vi "postCommandUserEvent.vi"(8 "error in (no error)":errorcluster, 10 "unsigned byte array":u8[](array[numeric]), 11 "DataListenerThisComponent in":refnum<class "DataListenerThisComponent.lvclass">) -> (0 "error out":errorcluster, 3 "DataListenerThisComponent out":refnum<class "DataListenerThisComponent.lvclass">)   [LabVIEW 2015, in "DataListenerThisComponent.lvclass"]
uses:
  DataListenerThisComponent.lvclass
  ComponentTemplateCore/ComponentModel/ComponentModel/DataListener/DataListener.lvclass/DataListener.ctl
  ComponentTemplateCore/ComponentModel/ComponentModel/CommandEvent/CommandEvent.lvclass/CommandEvent.ctl
  ComponentTemplateCore/ComponentModel/ComponentModel/CommandEvent/CommandEvent.lvclass
  ComponentTemplateCore/ComponentModel/ComponentModel/DataListener/DataListener.lvclass
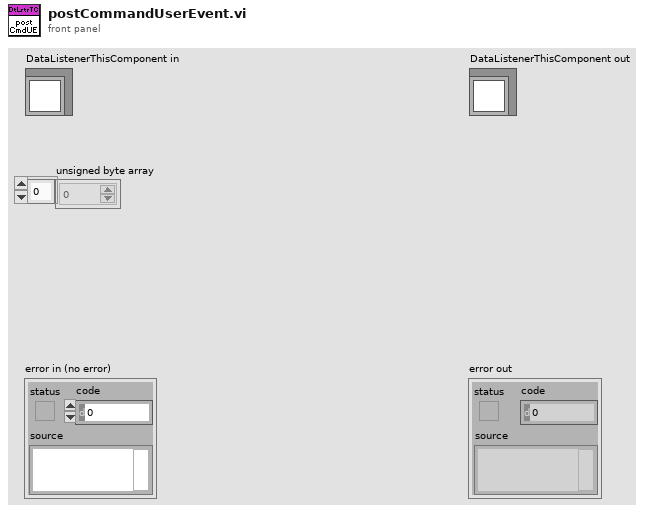
[diagram p1: front panel]
types:
  T1 = typedef "EXATypedefs.lvlib/CommandEvents.ctl" = cluster{"command":refnum<user-event>}
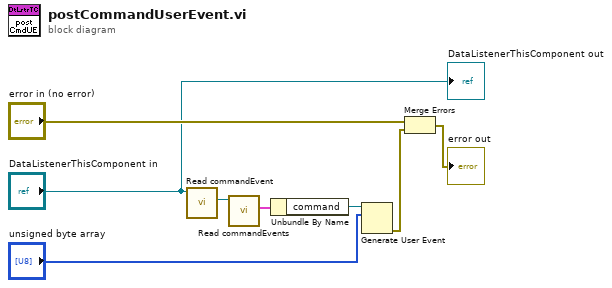
[diagram p0: block diagram]
diagram:
  n1 = call "Read commandEvent.vi"("DataListener in"="DataListenerThisComponent in") -> ("commandEvent"=w2:refnum<class "CommandEvent.lvclass">)  [unwired: 9 in, 1 out]
  n2 = call "Read commandEvents.vi"("CommandEvent in"=w2) -> ("CommandEvents"=w1:T1)  [unwired: 9 in, 1 out]
  n3 = Unbundle By Name(w1) -> ("command"=w8:refnum<user-event>)
  n4 = Generate User Event(user event=w8, event data cluster="unsigned byte array") -> (error out=w5:errorcluster)  [unwired: 2 in, 1 out]
  n5 = Merge Errors("error in (no error)", w5) -> (→"error out":errorcluster)
  "DataListenerThisComponent out" <- "DataListenerThisComponent in"
